vi "Create REST Client.vi"(4 "Default Headers ([JSON])":T1[](array[typedef])=[{"header"="Content-Type", "value"="application/json"}], 5 "REST Client in":refnum<class "REST Client.lvclass">, 6 "Verify Server(true)":bool=TRUE, 8 "error in (no error)":errorcluster, 10 "Escape URLs (true)":bool=TRUE, 11 "Base URL":string) -> (0 "error out":errorcluster, 3 "REST Client out":refnum<class "REST Client.lvclass">)   [LabVIEW 2018, in "REST Client_JKI.lvlib" / "REST Client.lvclass"]
doc: "The VI provides multiple arguments for defining how to create the JKI REST Client instance.\n\n<b>Base URL</b> specifies the base URL to be used for the HTTP requests.\n\n<b>Escape URLs</b> when true instruct the REST Client to escape all URLs before executing the requests. If you have already escaped the URLs, set this to false.\n\n<b>Authentication</b> allows setting the username and password for services that use HTTP authentication.\n\n<b>Verify Server</b> when true instructs the REST Client to validate the certificate of the server when HTTPS protocol is being used.\n\n<b>Default Headers</b> specifies an array of headers to be used with every requests. Defaults to application/json content type.\n\n<b>Cookie File</b> specifies a file path to be used for cookies."
uses:
  REST Client.lvclass
  HTTP Header.ctl
  REST Client.lvclass/REST Client.ctl
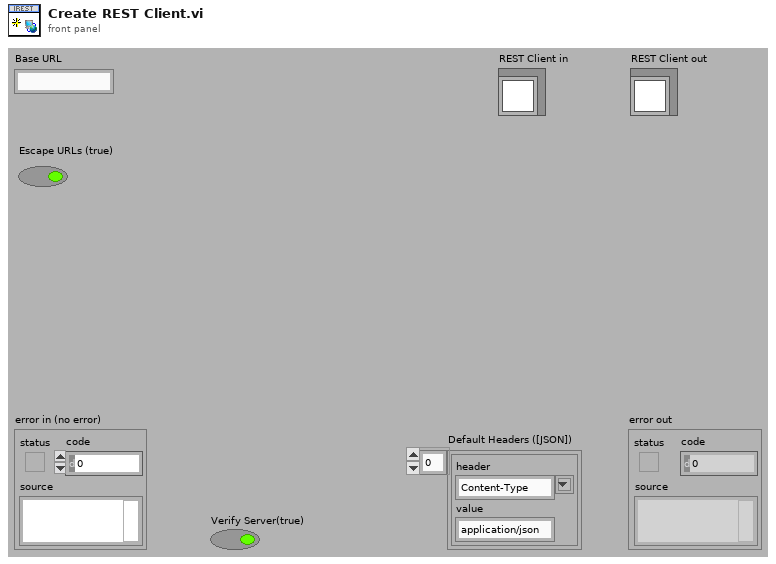
[diagram p1: front panel]
types:
  T1 = typedef "REST Client_JKI.lvlib/REST Client.lvclass/HTTP Header.ctl" = cluster{"header":string, "value":string}
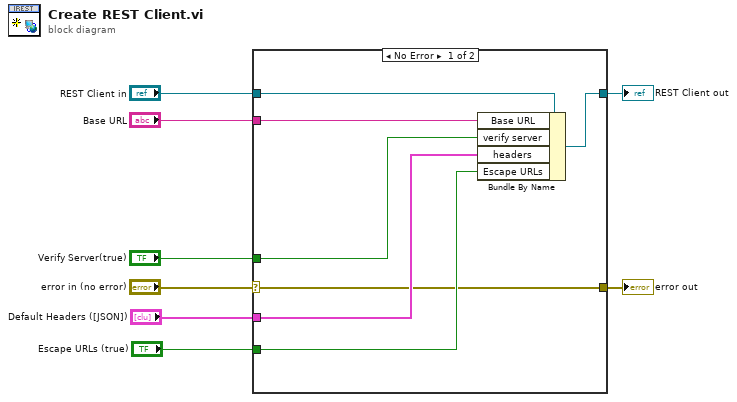
[diagram p0: block diagram]
diagram:
  n1 = case shown="No Error" "error in (no error)" {
    selector: "error in (no error)" -> [w9 w17]
    tunnel: [w9 w17] -> w7
    tunnel: [w15 w16] -> w5
    tunnel: "REST Client in" -> [w10 w16]
    tunnel: "Verify Server(true)" -> [w13 _]
    tunnel: "Default Headers ([JSON])" -> [w12 _]
    tunnel: "Base URL" -> [w14 _]
    tunnel: "Escape URLs (true)" -> [w11 _]
    frame No Error {
      n2 = Bundle By Name(cluster=w10, "Base URL"=w14, "verify server"=w13, "headers"=w12, "Escape URLs"=w11) -> (w15:refnum<class "REST Client.lvclass">)
    }
    frame Error {
    }
  }
  "error out" <- w7
  "REST Client out" <- w5
